vi "Rename as Application Name.vi"() -> ()   [LabVIEW 2020]
doc: "This VI can be used as a launcher VI for the main application or as a debugging tool.\n_____\nBased on DQMH Project Template 6.1.0.94."
uses:
  <vilib>/Utility/error.llb/DialogType.ctl
  Libraries/Launcher Support/Launcher Support.lvlib
  <vilib>/Peloton/Pelobuttons/Pelobuttons_lib_Pelobuttons.lvlib
  <vilib>/addons/_BLT for LabVIEW/BLT_SourceDistribution.llb/BLT_Spy.lvlib
  Libraries/Rename as Top-Level Library/Rename as Top-Level Library.lvlib
panel:
  in  "Launch API Tester":bool
  out "Command Line Arguments":string[](array[string])
  out "Module Running?":bool
  out "Status":string
  out "error out":errorcluster
  in  "Stop Module":bool
  in  "Start Module":bool
  # "Make sure you use Pelobuttons to edit your Main UI"
  # "See the Build_Final_EXE bookmarks on the diagram for instructions on using this VI as a launcher for an EXE."
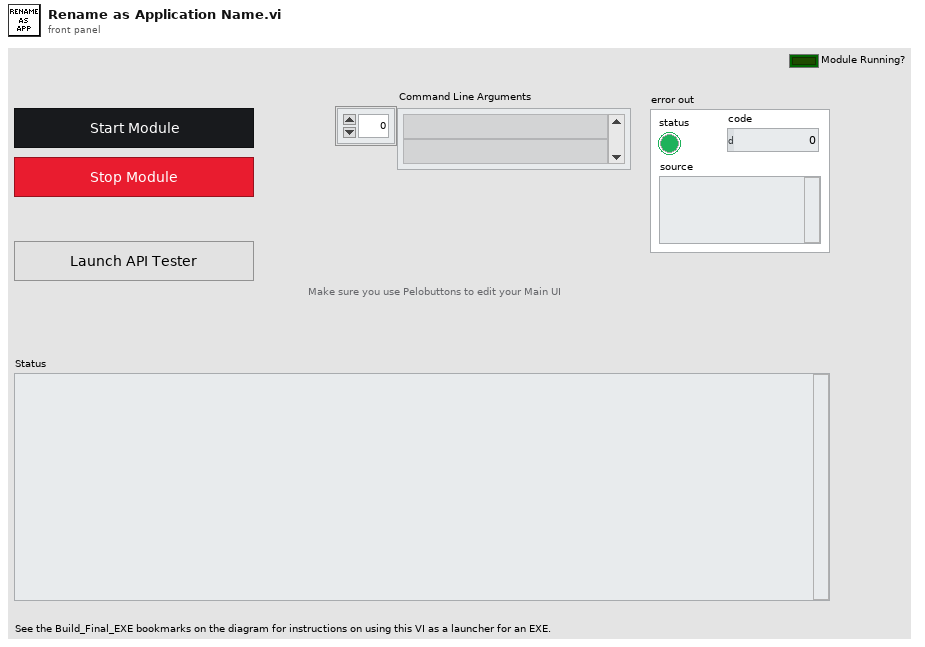
[diagram p1: front panel]
types:
  T1 = enum32{"invalid app kind", "Development System", "Run Time System", "Student Edition", "Embedded LabVIEW", "Evaluation", "Custom"}
  T2 = typedef "Rename as Top-Level Library.lvlib/Broadcast Events--cluster.ctl" = cluster{"Module Did Init":refnum<user-event>, "Status Updated":refnum<user-event>, "Error Reported":refnum<user-event>, "Module Did Stop":refnum<user-event>, "Update Module Execution Status":refnum<user-event>}
  T3 = typedef "DialogType.ctl" = u16
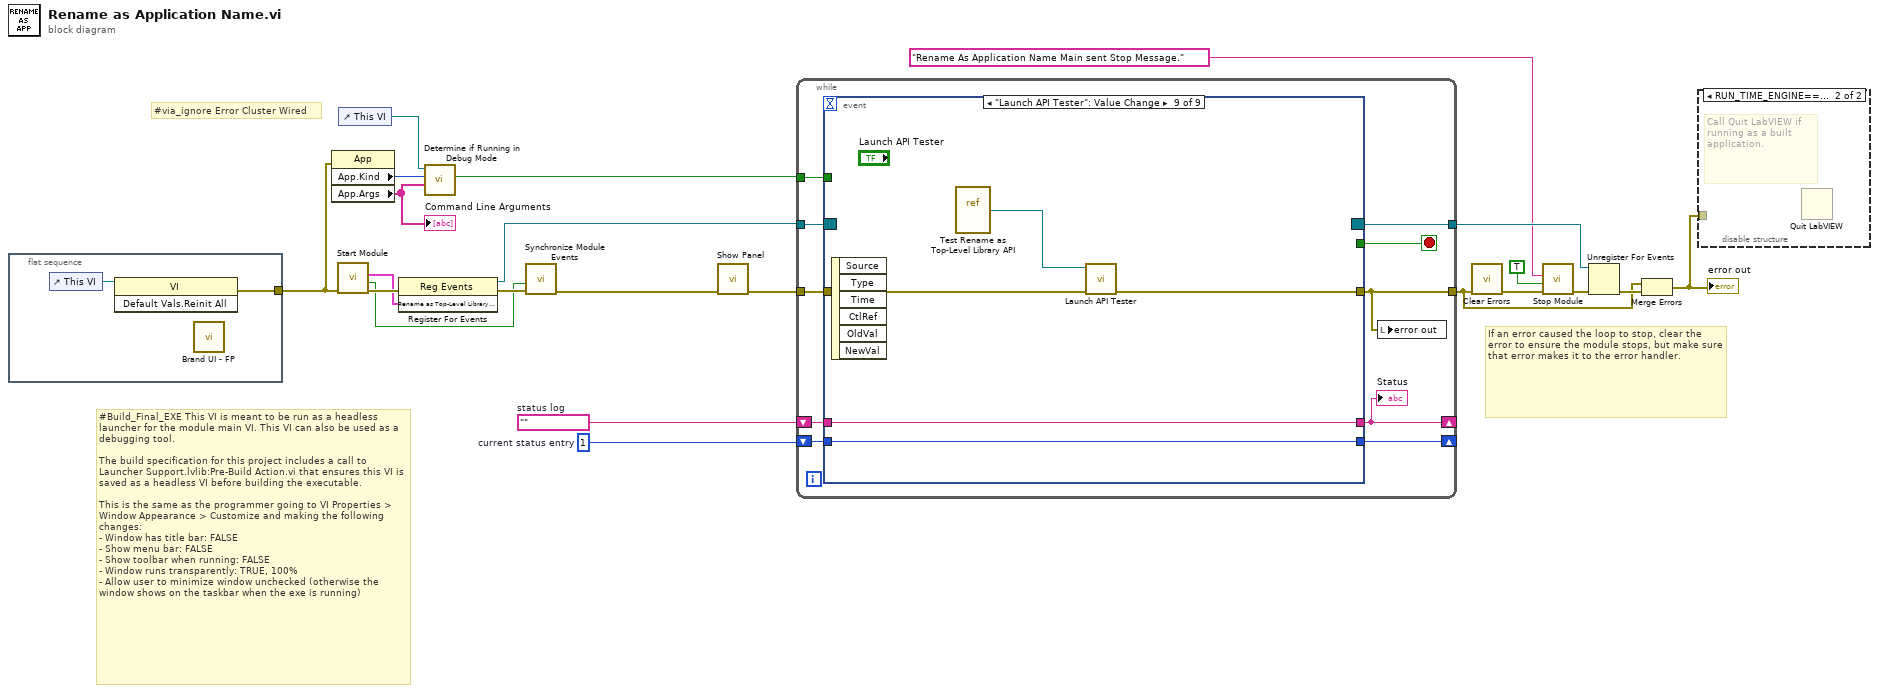
[diagram p0: block diagram]
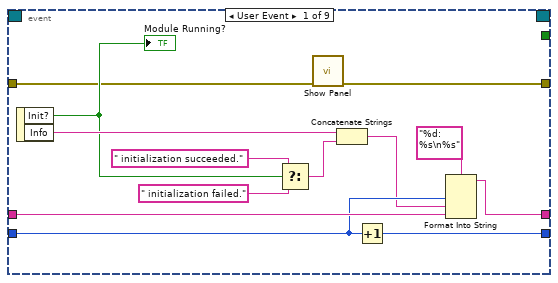
[diagram p2: hidden frame]
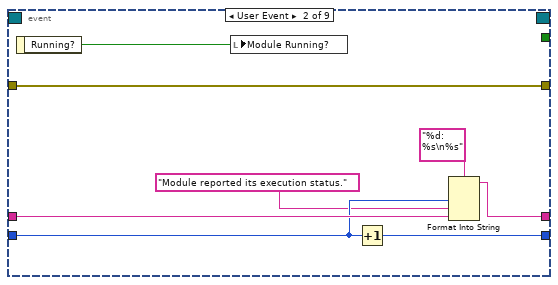
[diagram p3: hidden frame]
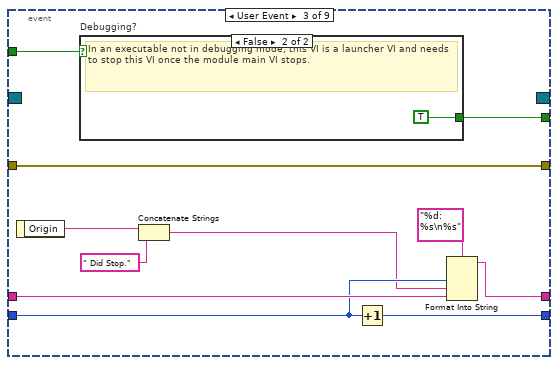
[diagram p4: hidden frame]
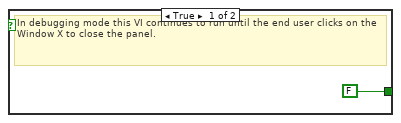
[diagram p5: hidden frame]
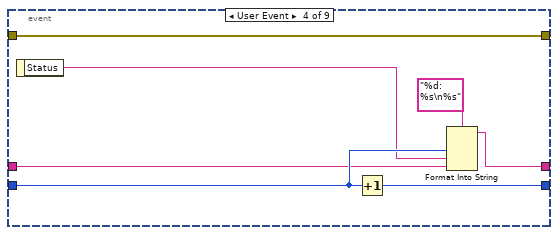
[diagram p6: hidden frame]
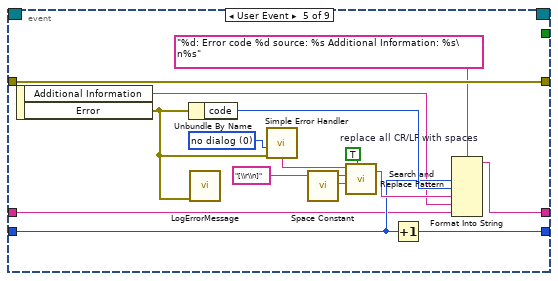
[diagram p7: hidden frame]
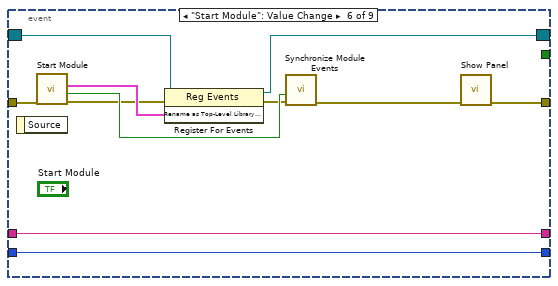
[diagram p8: hidden frame]
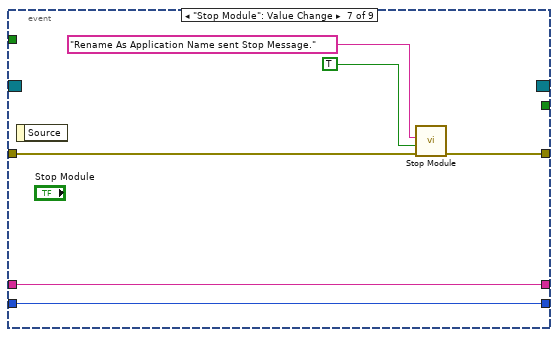
[diagram p9: hidden frame]
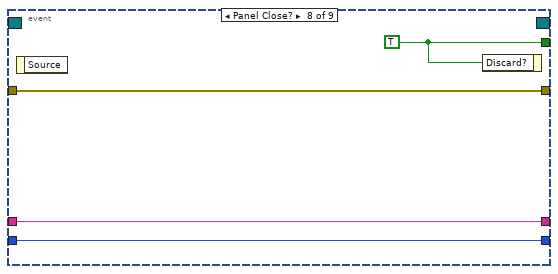
[diagram p10: hidden frame]
diagram:
  w20 = 1  # current status entry
  w21 = ""  # status log
  # "#via_ignore Error Cluster Wired"
  # "#Build_Final_EXE This VI is meant to be run as a headless launcher for the module main VI. This VI can also be used as a debugging tool. \n\nThe build specification for this project includes a call to Launcher Support.lvlib:Pre-Build Action.vi that ensures this VI is saved as a headless VI before building the executable.\n\nThis is the same as the programmer going to VI Properties > Window Appearance > Customize and making the following changes:\n- Window has title bar: FALSE\n- Show menu bar: FALSE\n- Show toolbar when running: FALSE\n- Window runs transparently: TRUE, 100%\n- Allow user to minimize window unchecked (otherwise the window shows on the taskbar when the exe is running)"
  # "If an error caused the loop to stop, clear the error to ensure the module stops, but make sure that error makes it to the error handler."
  n1 = flat-sequence {
    tunnel: [w24] -> w11
    frame #0 {
      n2 = control-ref of="This VI"() -> (w23:refnum<vi>)
      n3 = invoke on="Invoke Node" class="VI" method="Default Vals.Reinit All"(reference=w23) -> (error out=w24:errorcluster)  [unwired: 2 in, 2 out]
      n4 = call <vilib>:"Brand UI - FP.vi"() -> ()  [unwired: 12 in]
    }
  }
  n5 = property on="Property Node" class="App"(error in=w11) -> ("App.Kind"=w12:T1, "App.Args"=w15:string[])  [unwired: 1 in, 2 out]
  "Command Line Arguments" <- w15
  n6 = call "Start Module.vi"("error in"=w11) -> ("error out"=w10:errorcluster, "Wait for Event Sync?"=w7:bool, "Rename as Top-Level Library Broadcast Events"=w9:T2)  [unwired: 7 in, 1 out]
  n7 = control-ref of="This VI"() -> (w14:refnum<vi>)
  n8 = register-events(error in=w10, w9) -> (reference out=w18:refnum<event-registration>, error out=w8:errorcluster)  [unwired: 1 in]
  n9 = call "Determine if Running in Debug Mode.vi"("App.Args"=w15, "App.Kind"=w12, "Launcher VI ref"=w14) -> ("Debug mode?"=w13:bool)  [unwired: 8 in]
  n10 = call "Synchronize Module Events.vi"("error in"=w8, "Wait for Event Sync?"=w7) -> ("error out"=w2:errorcluster)  [unwired: 9 in]
  n11 = call "Show Panel.vi"("error in (no error)"=w2) -> ("error out"=w1:errorcluster)  [unwired: 10 in]
  n12 = while {
    tunnel: w18 -> [w34]
    tunnel: [w26] -> w16
    shift-right: [w27] -> _
    shift-left: w21 -> [w31]
    shift-right: [w30] -> _
    shift-left: w20 -> [w32]
    tunnel: w1 -> [w29]
    tunnel: [w28] -> w19
    tunnel: w13 -> [w25]
    stop <- w33 stop-if-true
    n13 = event shown="[8] \"Launch API Tester\": Value Change" {
      selector: w34 -> [_ _ _ _ _ w92 _ _ _]
      dyn-events: [_ _ _ _ _ w91 _ _ _] -> w28
      timeout: _ -> [_ _ _ _ _ _ _ _ _]
      tunnel: [_ _ w57 _ _ _ _ w111 _] -> w33
      tunnel: [w35 w49 w58 w69 w90 w93 w103 w108 w113] -> w26
      tunnel: w32 -> [w45 w53 w64 w72 w82 w100 w106 w109 w115]
      tunnel: w31 -> [w46 w54 w65 w71 w80 w101 w107 w110 w116]
      tunnel: [w43 w51 w62 w73 w83 w101 w107 w110 w116] -> w27
      tunnel: [w44 w52 w63 w75 w81 w100 w106 w109 w115] -> w30
      tunnel: w29 -> [w36 w49 w58 w69 w90 w95 w104 w108 w112]
      tunnel: w25 -> [_ _ w56 _ _ _ _ _ _]
      event User Event {
        n14 = event-data() -> ("Init?"=w40:bool, "Info"=w42:string)  [unwired: 1 in]
        "Module Running?" <- w40
        n15 = Select(t=" initialization succeeded.", s=w40, f=" initialization failed.") -> (s? t:f=w37:string)
        n16 = call "Show Panel.vi"("error in (no error)"=w36) -> ("error out"=w35:errorcluster)  [unwired: 10 in]
        n17 = Concatenate Strings(w42, w37) -> (w41:string)
        n18 = Increment(x=w45) -> (x+1=w44:i32)
        n19 = Format Into String(format string="%d: %s\n%s", w45, w41, w46) -> (resulting string=w43:string)  [unwired: 2 in, 1 out]
      }
      event User Event {
        n20 = event-data() -> ("Running?"=w48:bool)  [unwired: 1 in]
        n21 = local write "Module Running?"(w48) -> ()
        n22 = Increment(x=w53) -> (x+1=w52:i32)
        n23 = Format Into String(format string="%d: %s\n%s", w53, "Module reported its execution status.", w54) -> (resulting string=w51:string)  [unwired: 2 in, 1 out]
      }
      event User Event {
        n24 = event-data() -> ("Origin"=w61:string)  [unwired: 1 in]
        n25 = case "Debugging?" shown="False" w56 {
          tunnel: [FALSE ("Discard?") TRUE ("Discard?")] -> w57
          frame True {
            # "In debugging mode this VI continues to run until the end user clicks on the Window X to close the panel."
          }
          frame False {
            # "In an executable not in debugging mode, this VI is a launcher VI and needs to stop this VI once the module main VI stops."
          }
        }
        n26 = Concatenate Strings(w61, " Did Stop.") -> (w60:string)
        n27 = Increment(x=w64) -> (x+1=w63:i32)
        n28 = Format Into String(format string="%d: %s\n%s", w64, w60, w65) -> (resulting string=w62:string)  [unwired: 2 in, 1 out]
      }
      event User Event {
        n29 = event-data() -> ("Status"=w70:string)  [unwired: 1 in]
        n30 = Increment(x=w72) -> (x+1=w75:i32)
        n31 = Format Into String(format string="%d: %s\n%s", w72, w70, w71) -> (resulting string=w73:string)  [unwired: 2 in, 1 out]
      }
      event User Event {
        w78 = T3 0 items=["no dialog", "OK message", "continue or stop message", "OK message + warnings", "continue/stop + warnings"] ("type of dialog (OK msg:1)")
        w86 = TRUE  # replace all CR/LF with spaces
        n32 = event-data() -> ("Additional Information"=w79:string, "Error"=w77:errorcluster)  [unwired: 1 in]
        n33 = Unbundle By Name(w77) -> ("code"=w84:i32)
        n34 = call <vilib>:"LogErrorMessage.vi"("error in (no error)"=w77) -> ()  [unwired: 10 in, 1 out]
        n35 = call <vilib>:"Simple Error Handler.vi"("type of dialog (OK msg:1)"=w78, "error in (no error)"=w77) -> ("message"=w76:string)  [unwired: 3 in, 4 out]
        n36 = call <vilib>:"Space Constant.vi"() -> ("String"=w87:string)
        n37 = call <vilib>:"Search and Replace Pattern.vi"("string"=w76, "regular expression (\"\")"="[\\r\\n]" ("regular expression (\"\")"), "replace string (\"\")"=w87, "replace all? (F)"=w86) -> ("result string"=w85:string)  [unwired: 1 in, 1 out]
        n38 = Increment(x=w82) -> (x+1=w81:i32)
        n39 = Format Into String(format string="%d: Error code %d source: %s Additional Information: %s\n%s", w82, w84, w85, w79, w80) -> (resulting string=w83:string)  [unwired: 2 in, 1 out]
      }
      event "Start Module": Value Change {
        n40 = event-data() -> ()  [unwired: 1 in, 1 out]
        n41 = call "Start Module.vi"("error in"=w95) -> ("error out"=w96:errorcluster, "Wait for Event Sync?"=w99:bool, "Rename as Top-Level Library Broadcast Events"=w97:T2)  [unwired: 7 in, 1 out]
        n42 = register-events(reference=w92, error in=w96, w97) -> (reference out=w91:refnum<event-registration>, error out=w98:errorcluster)
        n43 = call "Synchronize Module Events.vi"("error in"=w98, "Wait for Event Sync?"=w99) -> ("error out"=w94:errorcluster)  [unwired: 9 in]
        n44 = call "Show Panel.vi"("error in (no error)"=w94) -> ("error out"=w93:errorcluster)  [unwired: 10 in]
      }
      event "Stop Module": Value Change {
        n45 = event-data() -> ()  [unwired: 1 in, 1 out]
        n46 = call "Stop Module.vi"("error in"=w104, "Wait for Module to Stop? (F)"=TRUE, "Origin"="Rename As Application Name sent Stop Message.") -> ("error out"=w103:errorcluster)  [unwired: 8 in]
      }
      event Panel Close? {
        w111 = TRUE ("Discard?")
        n47 = event-data() -> ()  [unwired: 1 in, 1 out]
        n48 = event-data ("Event Filter Node")("Discard?"=w111) -> ()  [unwired: 1 in, 1 out]
      }
      event "Launch API Tester": Value Change {
        n49 = event-data() -> ()  [unwired: 1 in, 6 out]
        n50 = vi-ref "Test Rename as Top-Level Library API.vi"() -> (w114:refnum<vi>)
        n51 = call "Launch API Tester.vi"("error in"=w112, "VI in"=w114) -> ("error out"=w113:errorcluster)  [unwired: 9 in]
      }
    }
    "Status" <- w27
    n52 = local write "error out"(w26) -> ()
  }
  n53 = call <vilib>:"Clear Errors.vi"("error in (no error)"=w16) -> ("error out"=w6:errorcluster)  [unwired: 5 in, 1 out]
  n54 = call "Stop Module.vi"("error in"=w6, "Wait for Module to Stop? (F)"=TRUE ("Wait for Module to stop?"), "Origin"="Rename As Application Name Main sent Stop Message.") -> ("error out"=w5:errorcluster)  [unwired: 8 in]
  n55 = Unregister For Events(event registration refnum=w19, error in=w5) -> (error out=w22:errorcluster)
  n56 = Merge Errors(w16, w22) -> (w17:errorcluster)
  "error out" <- w17
  n57 = disable-structure "Conditional Disable Structure" shown="RUN_TIME_ENGINE==True" {
    disable-tunnel: w17 -> [_ _]
    frame condition #0 (active) {
    }
    frame condition #1 {
      # "Call Quit LabVIEW if running as a built application."
      n58 = Quit LabVIEW() -> ()  [unwired: 1 in]
    }
  }
